vi "Food Truck Main.vi"() -> ()   [LabVIEW 2013]
doc: "This example shows how to debounce a digital signal acquired from a push button switch."
uses:
  <vilib>/Platform/TimedLoop/XDataNode/timing_clust.ctl
  <vilib>/Platform/TimedLoop/XDataNode/nitl_modes.ctl
  <vilib>/Platform/TimedLoop/XDataNode/wakeup.ctl
  Controls/ATT M2X Streams.ctl
  <vilib>/myRIO/Instrument Drivers/Onboard IO/AI/vis/Smart Open.vi
  <vilib>/myRIO/Instrument Drivers/Onboard IO/AI/vis/Read.vi
  <vilib>/myRIO/Instrument Drivers/Onboard IO/DIO/vis/Smart Open.vi
  <vilib>/myRIO/Instrument Drivers/Onboard IO/DIO/vis/Read.vi
  <vilib>/myRIO/Common/Instrument Driver Framework/myRIO v1.0/UART/vis/myRIO v1.0 Close UART.vi
  <vilib>/myRIO/Instrument Drivers/Onboard IO/AI/vis/Open.vi
  <vilib>/myRIO/Instrument Drivers/Onboard IO/DIO/vis/Open.vi
  <vilib>/myRIO/Common/Instrument Driver Framework/myRIO v1.0/AI/vis/myRIO v1.1 Open AI.vi
  <vilib>/myRIO/Common/Instrument Driver Framework/myRIO v1.0/DIO/vis/myRIO v1.1 Open DIO.vi
  <vilib>/myRIO/Common/Instrument Driver Framework/Utilities/vis/Validate Channels.vi
  <vilib>/myRIO/Common/Instrument Driver Framework/myRIO v1.0/AI/vis/myRIO v1.0 Reserve AI.vi
  <vilib>/myRIO/Common/Instrument Driver Framework/myRIO v1.0/DIO/vis/myRIO v1.0 Reserve DIO.vi
  <vilib>/myRIO/Common/Instrument Driver Framework/myRIO v1.0/AI/vis/myRIO v1.0 Build MUX Configuration AI.vi
  <vilib>/myRIO/Common/Instrument Driver Framework/myRIO v1.0/Resource Manager/vis/myRIO v1.0 Reserve Channel List.vi
  <vilib>/myRIO/Common/Instrument Driver Framework/myRIO v1.0/DIO/vis/myRIO v1.0 Build MUX Configuration DIO.vi
  <vilib>/myRIO/Common/Instrument Driver Framework/myRIO v1.0/Resource Manager/vis/myRIO v1.0 Reserve Channel.vi
  <vilib>/myRIO/Common/Instrument Driver Framework/myRIO v1.0/Resource Manager/vis/myRIO v1.0 Unreserve Channel.vi
  <vilib>/myRIO/Common/Instrument Driver Framework/myRIO v1.0/Resource Manager/vis/myRIO v1.0 Create Configuration List.vi
  <vilib>/myRIO/Common/Instrument Driver Framework/myRIO v1.0/Resource Manager/vis/myRIO v1.0 Build Mutex Name.vi
  <vilib>/Instr/_visa.llb/VISA Configure Serial Port (Instr).vi
  <vilib>/myRIO/Common/Instrument Driver Framework/myRIO v1.0/myRIO v1.1 Open.vi
  <vilib>/myRIO/Common/Instrument Driver Framework/myRIO v1.0/AI/vis/myRIO v1.0 Get Scaling Constants AI.vi
  <vilib>/Utility/VariantDataType/GetNumericInfo.vi
  <vilib>/Utility/error.llb/Error Cluster From Error Code.vi
  <vilib>/myRIO/Common/Instrument Driver Framework/Utilities/vis/IO Manager.vi
  <vilib>/myRIO/Common/Instrument Driver Framework/Utilities/vis/Configuration Manager.vi
  <vilib>/myRIO/Common/Instrument Driver Framework/myRIO v1.0/myRIO v1.0 Close.vi
  <vilib>/myRIO/Common/Instrument Driver Framework/myRIO v1.0/AI/vis/myRIO v1.0 Read AI.vi
  <vilib>/LVH/i3 Twitter/SubVIs/Twitter Open - Embedded.vi
  <vilib>/myRIO/Common/Instrument Driver Framework/myRIO v1.0/Resource Manager/vis/myRIO v1.0 Configure IO.vi
  <vilib>/myRIO/Common/Instrument Driver Framework/myRIO v1.0/DIO/vis/myRIO v1.0 Read DIO.vi
  <vilib>/myRIO/Common/Instrument Driver Framework/Utilities/vis/FPGA Ref Manager.vi
  <vilib>/myRIO/Common/Instrument Driver Framework/myRIO v1.0/myRIO v1.0 Reset FPGA.vi
  <vilib>/Platform/TimedLoop/XDataNode/XDataNode.xnode
  <vilib>/Platform/TimedLoop/XDataNode/XDNodeRunTimeDep.lvlib
  <vilib>/LVH/i3 Twitter/i3-twitter.lvlib
  <vilib>/myRIO/Instrument Drivers/Utilities/Utilities.lvlib
panel:
  out "Current Sunshine Value":dbl
  out "Current Food Temp (F)":dbl
  out "Food and Sunshine Timer (30s)":dbl
  out "GPS Timer (180s)":dbl
  out "Latest GPS Transit Data":string
  out "Button Clicks":u16(graph)
  in  "Send to Servers":bool=TRUE
  out "error out":errorcluster
  in  "Stop":bool
  # "Overview: This example shows how to debounce a digital signal acquired from a push button switch.\nInstructions:\n1. Connect an external push button switch to DIO0 on connector A.\n2. Check the myRIO target IP Address in the project and make sure the target IP Address is correct.\n3. Run this VI.\n4. Depending on the quality of the push button switch, you may or may not see jitter."
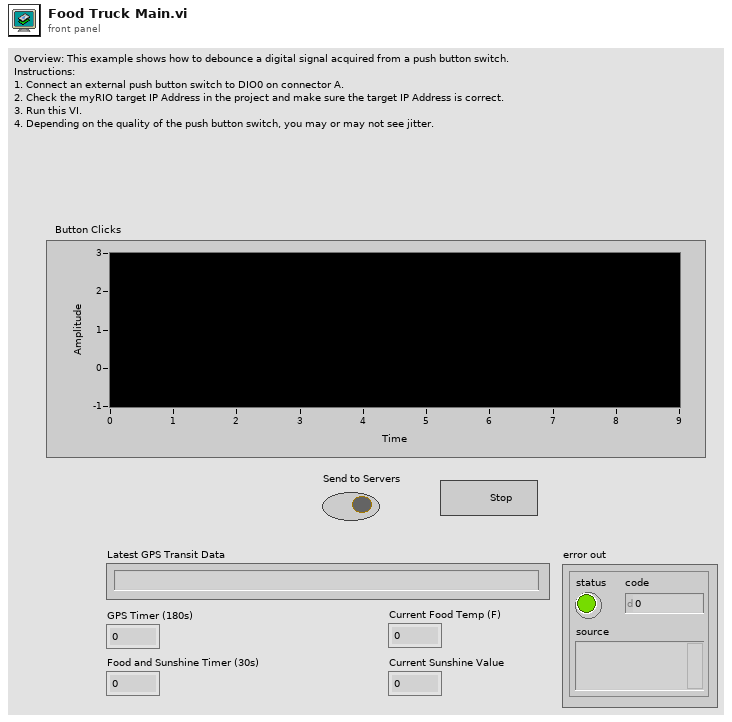
[diagram p1: front panel]
types:
  T1 = cluster{"read mode":enum16{"polling", "blocking"}, "write mode":enum16{"polling", "blocking"}}
  T2 = typedef "ATT M2X Streams.ctl" = enum16{"pay", "deliver", "sunshine", "location", "temp"}
  T3 = typedef "XDNodeRunTimeDep.lvlib/timing_clust.ctl" = cluster{"Expected End [f-1]":u64, "Actual End [f-1]":u64, "Finished Late? [f-1]":bool, "Expected End [i-1]":u64, "Actual End [i-1]":u64, "Finished Late? [i-1]":bool, "Expected Start [i]":u64, "Actual Start [i]":u64, "Expected Start [f]":u64, "Actual Start [f]":u64, "Source Name":string, "Structure Name":string, "Period":i64, "Deadline":i64, "Offset":i64, "Start":i64, "Priority":i32, "Timeout":i32, "Mode":T4, "Wakeup Reason":T5, "Error":errorcluster, "Source Type":string, "Secondary Source Type":string, "Global End Time":u64, "Global Start Time":u64, "Frame Duration":u64, "Iteration Duration":u64, "Assigned CPU":i32, "I/O Scan Engine Mode":u32}
  T4 = typedef "XDNodeRunTimeDep.lvlib/nitl_modes.ctl" = enum32{"No Change", "Process missed periods, maintain original phase", "Discard missed periods, maintain original phase", "Process missed periods, ignore original phase", "Discard missed periods, ignore original phase"}
  T5 = typedef "XDNodeRunTimeDep.lvlib/wakeup.ctl" = enum32{"Normal", "Aborted", "Asynchronous wakeup", "Timing source error", "Timed loop error", "Timeout"}
  T6 = typedef "IMAQ Image.ctl" = refnum<image>
  T7 = typedef "i3-twitter.lvlib/Twitter Handle.ctl" = cluster{"OAuth Credentials":T8, "since ID":string, "max ID":string, "Screen Name":string}
  T8 = typedef "i3-oauth.lvlib/OAuth Handle.ctl" = cluster{"Signature Method":T9, "Version":string, "Client":T10, "Access":T10}
  T9 = typedef "i3-oauth.lvlib/Signature Method.ctl" = enum16{"HMAC-MD5", "HMAC-SHA1", "HMAC-SHA224", "HMAC-SHA256", "HMAC-SHA384", "HMAC-SHA512"}
  T10 = typedef "i3-oauth.lvlib/Credentials.ctl" = cluster{"Token":string, "Secret":string}
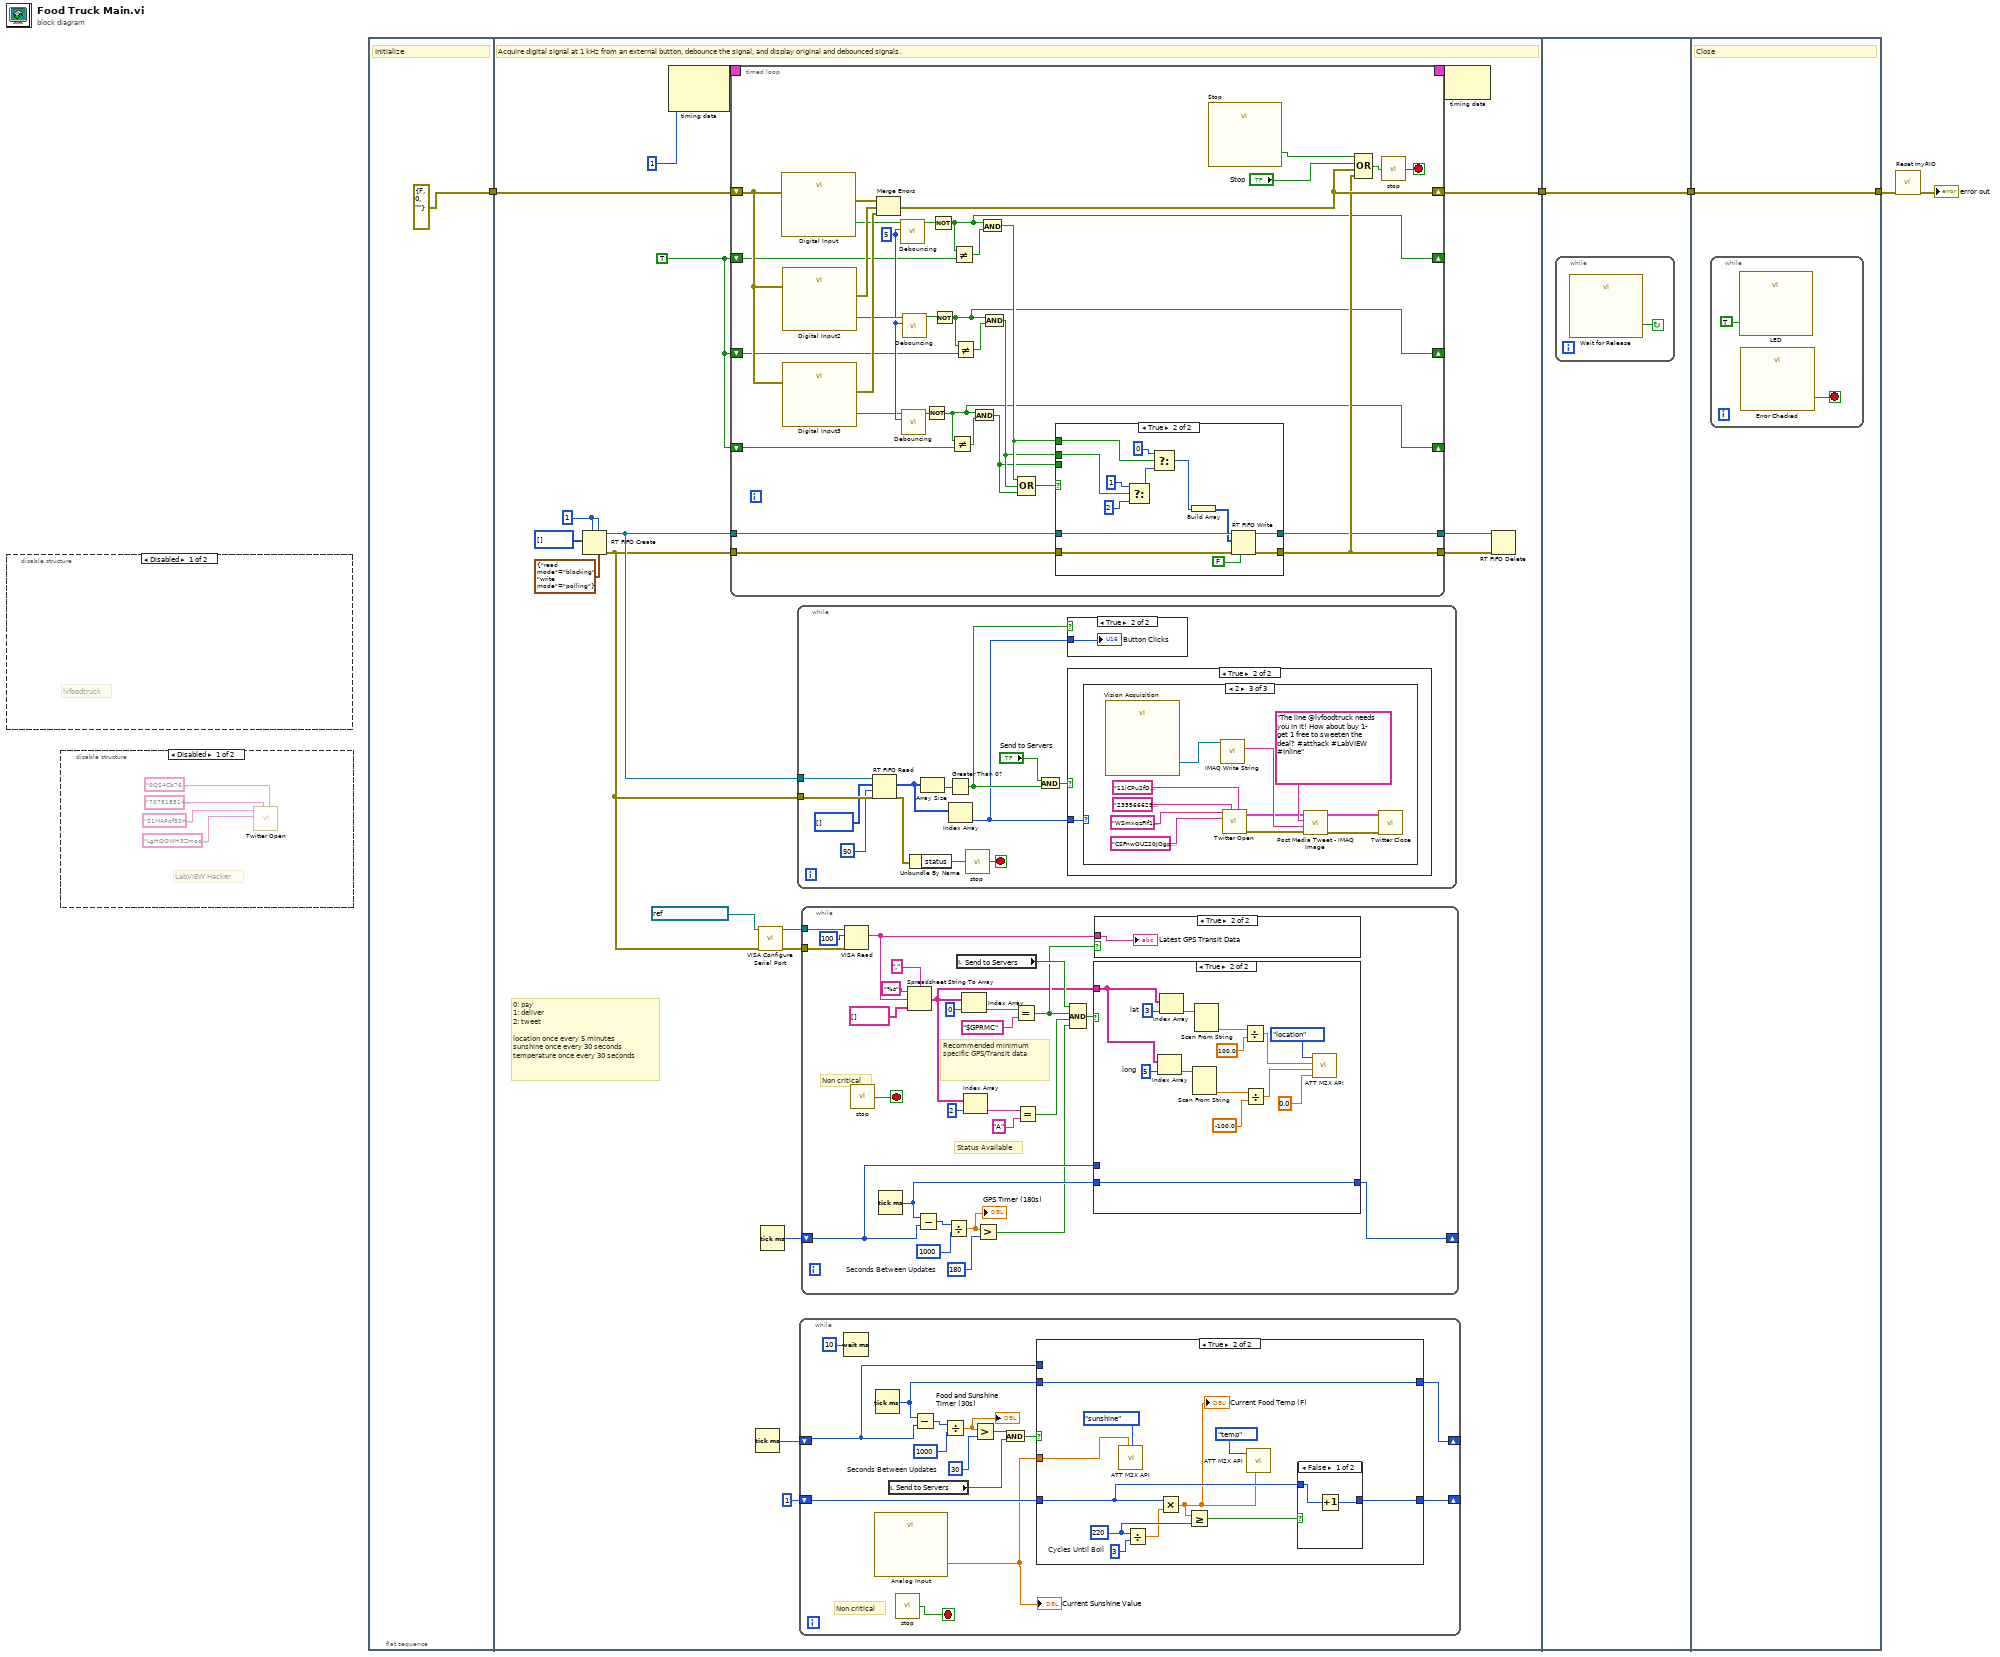
[diagram p0: block diagram]
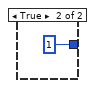
[diagram p5: hidden frame]
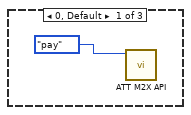
[diagram p10: hidden frame]
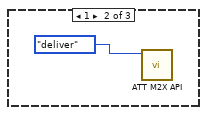
[diagram p11: hidden frame]
diagram:
  n1 = disable-structure shown="Disabled" {
    frame Disabled {
      # "lvfoodtruck"
    }
    frame Enabled {
    }
  }
  n2 = disable-structure shown="Disabled" {
    frame Disabled {
      # "LabVIEW Hacker"
      n3 = call-poly <vilib>:"Twitter Open.vi"("Access Secret"="0QS4Cb76M5wjFwPQ7tOZFvZ8UKrVkLlgPVmxGdh9fF0", "Access Token"="707518514-5GkAQhxzcTAC2kfWjk70QnGtfbYQtNPzzYrLQPwE", "Consumer Secret"="LgHQOWH3ZmoqpZxo5fXh4u8m0SzKCa7qTMPE3lom3I", "Consumer Key"="S1MAPof5SHW02X1IO2gQkA") -> ()  [unwired: 6 in, 2 out]
    }
    frame Enabled {
    }
  }
  n4 = flat-sequence {
    tunnel: [errorcluster {"status"=FALSE, "code"=0, "source"=""} ("error out")] -> w5
    tunnel: w5 -> [w27]
    tunnel: [w26] -> w2
    tunnel: w2 -> [w186]
    tunnel: [w186] -> w1
    tunnel: w1 -> [w188]
    tunnel: [w188] -> w4
    frame #0 {
      # "Initialize"
    }
    frame #1 {
      w18 = TRUE ("A/DIO0 (Pin 11)")
      w24 = u32 1 ("size (10)")
      # "0: pay\n1: deliver\n2: tweet\n\nlocation once every 5 minutes\nsunshine once every 30 seconds\ntemperature once every 30 seconds"
      # "Acquire digital signal at 1 kHz from an external button, debounce the signal, and display original and debounced signals."
      n5 = RT FIFO Create(1:u16[] [], 4:w24, 6:w24, 7:T1 {"read mode"=enum."blocking", "write mode"=enum."polling"} ("r/w modes (polling,polling)")) -> (8:w22:refnum<k33>, 11:w17:errorcluster)  [unwired: 4 in, 1 out]
      n6 = node-c288(i64 1 ("Period")) -> (w29:T3)  [unwired: 1 in]
      n7 = timed-loop {
        shift-right: [w155] -> w26
        shift-left: w27 -> [w157]
        timing: w29 -> [_]
        timing-out: [_] -> w28
        tunnel: w22 -> [w152]
        tunnel: w17 -> [w153]
        tunnel: [w151] -> w19
        tunnel: [w150] -> w20
        shift-right: [w144] -> _
        shift-left: w18 -> [w146]
        shift-right: [w140] -> _
        shift-left: w18 -> [w139]
        shift-right: [w135] -> _
        shift-left: w18 -> [w136]
        stop <- w133 stop-if-true
        w159 = u16 5 ("Cycles to Filter")
        n8 = call "Digital Input"("error in (no error)"=w157) -> ("A/DIO0 (Pin 11)"=w161:bool, "error out"=w156:errorcluster)  [unwired: 25 in]
        n9 = call "Digital Input2"("error in (no error)"=w157) -> ("A/DIO1 (Pin 13)"=w160:bool, "error out"=w164:errorcluster)  [unwired: 25 in]
        n10 = call "Digital Input3"("error in (no error)"=w157) -> ("A/DIO2 (Pin 15)"=w158:bool, "error out"=w163:errorcluster)  [unwired: 25 in]
        n11 = Merge Errors(w156, w164, w163) -> (w155:errorcluster)
        n12 = call "Debouncing.vi"("Cycles to Filter"=w159, "New Input Signal"=w161) -> ("New Signal"=w149:bool)  [unwired: 8 in, 1 out]
        n13 = call "Debouncing.vi"("Cycles to Filter"=w159, "New Input Signal"=w158) -> ("New Signal"=w148:bool)  [unwired: 8 in, 1 out]
        n14 = call "Debouncing.vi"("Cycles to Filter"=w159, "New Input Signal"=w160) -> ("New Signal"=w142:bool)  [unwired: 8 in, 1 out]
        n15 = Not(x=w148) -> (.not. x?=w135:bool)
        n16 = Not(x=w149) -> (.not. x?=w144:bool)
        n17 = Not(x=w142) -> (.not. x?=w140:bool)
        n18 = Not Equal?(x=w135, y=w136) -> (x != y?=w138:bool)
        n19 = Not Equal?(x=w144, y=w146) -> (x != y?=w145:bool)
        n20 = Not Equal?(x=w140, y=w139) -> (x != y?=w143:bool)
        n21 = And(x=w135, y=w138) -> (x .and. y?=w137:bool)
        n22 = And(x=w144, y=w145) -> (x .and. y?=w147:bool)
        n23 = And(x=w140, y=w143) -> (x .and. y?=w141:bool)
        n24 = Compound Arithmetic op=OR(w147, w141, w137) -> (w154:bool)
        n25 = case shown="True" w154 {
          tunnel: w137 -> [_ _]
          tunnel: w141 -> [_ w176]
          tunnel: w147 -> [_ w179]
          tunnel: w153 -> [w165 w173]
          tunnel: w152 -> [w166 w172]
          tunnel: [w165 w170] -> w151
          tunnel: [w166 w169] -> w150
          frame False {
          }
          frame True {
            n26 = Select(t=u16 1 ("size (10)"), s=w176, f=u16 2 ("size (10)")) -> (s? t:f=w177:u16)
            n27 = Select(t=u16 0 ("size (10)"), s=w179, f=w177) -> (s? t:f=w168:u16)
            n28 = Build Array(w168) -> (w167:u16[])
            n29 = RT FIFO Write(0:w172, 1:w167, 3:w173, 5:FALSE ("overwrite on timeout (T)")) -> (8:w169:refnum<k33>, 11:w170:errorcluster)  [unwired: 1 in, 2 out]
          }
        }
        n30 = call "Stop"() -> ("Value"=w132:bool)  [unwired: 26 in, 1 out]
        n31 = Compound Arithmetic op=OR(w132, "Stop", w155, w151) -> (w134:bool)
        n32 = call "stop.vi"("Stop?"=w134) -> ("Stop Called"=w133:bool)
      }
      n33 = Tick Count (ms)() -> (millisecond timer value=w12:u32)
      n34 = call-poly "VISA Configure Serial Port"("VISA resource name"=refnum<visa-resource-name> "ASRL1::INSTR", "error in (no error)"=w17) -> ("VISA resource name out"=w14:refnum<visa-resource-name>, "error out"=w15:errorcluster)  [unwired: 12 in]
      n35 = Tick Count (ms)() -> (millisecond timer value=w13:u32)
      n36 = while {
        tunnel: w22 -> [w116]
        tunnel: w17 -> [w115]
        stop <- w105 stop-if-true
        n37 = RT FIFO Read(0:w116, 1:u16[] [], 2:50 ("timeout in ms (0)"), 3:w115) -> (9:w111:u16[], 11:w106:errorcluster)  [unwired: 3 out]
        n38 = Unbundle By Name(w106) -> ("status"=w104:bool)
        n39 = Array Size(array=w111) -> (size(s)=w112:i32)
        n40 = Greater Than 0?(x=w112) -> (x > 0?=w108:bool)
        n41 = Index Array(array=w111) -> (element=w107:u16)  [unwired: 1 in]
        n42 = call "stop.vi"("Stop?"=w104) -> ("Stop Called"=w105:bool)
        n43 = And(x="Send to Servers", y=w108) -> (x .and. y?=w110:bool)
        n44 = case shown="True" w108 {
          tunnel: w107 -> [_ w117]
          frame False {
          }
          frame True {
            "Button Clicks" <- w117
          }
        }
        n45 = case shown="True" w110 {
          tunnel: w107 -> [_ w118]
          frame False {
          }
          frame True {
            n46 = case shown="2" w118 {
              frame 0, Default {
                n47 = call "ATT M2X API.vi"("M2X Action"=ATT_M2X_Streams."pay") -> ()  [unwired: 11 in]
              }
              frame 1 {
                n48 = call "ATT M2X API.vi"("M2X Action"=ATT_M2X_Streams."deliver") -> ()  [unwired: 11 in]
              }
              frame 2 {
                n49 = call "Vision Acquisition"() -> ("Image Out"=w128:T6)  [unwired: 1 in, 26 out]
                n50 = call-poly "IMAQ Write String"("Image"=w128) -> ("FileString"=w127:string)  [unwired: 8 in, 2 out]
                n51 = call-poly <vilib>:"Twitter Open.vi"("Access Secret"="11iCPu2fD6roKbZOZ3n06jO3pBqYyJw5qbVKj0QqDCqT4", "Access Token"="2355666296-oROjxw2YO7ZtzIdD03PYHHbLc9t4A0mUO1yUdhK", "Consumer Secret"="CSFnwOUZ20JOgpVWiaVuvtkmC6NybXKYc1vpgfGJEs", "Consumer Key"="WSmxqzFIf1JXEhfN34MA") -> ("error out"=w122:errorcluster, "Twitter Handle Out"=w121:T7)  [unwired: 6 in]
                n52 = call "Post Media Tweet - IMAQ Image.vi"("error in"=w122, "PNG String"=w127, "Tweet"="The line @lvfoodtruck needs you in it! How about buy 1- get 1 free to sweeten the deal? #atthack #LabVIEW #Inline", "Twitter Handle In"=w121) -> ("error out"=w130:errorcluster, "Twitter Handle Out"=w129:T7)  [unwired: 6 in]
                n53 = call <vilib>:"Twitter Close.vi"("error in"=w130, "Twitter Handle In"=w129) -> ()  [unwired: 9 in, 1 out]
              }
            }
          }
        }
      }
      n54 = while {
        shift-right: [w37] -> _
        shift-left: w12 -> [w38]
        shift-right: [w34] -> _
        shift-left: u32 1 ("y") -> [w35]
        stop <- w44 stop-if-true
        w43 = u32 30  # Seconds Between Updates
        # "Non critical"
        n55 = Wait (ms)(milliseconds to wait=u32 10) -> ()  [unwired: 1 out]
        n56 = call "Analog Input"() -> ("Sunshine (A/AI0 (Pin 3))"=w30:dbl)  [unwired: 26 in, 1 out]
        "Current Sunshine Value" <- w30
        n57 = Tick Count (ms)() -> (millisecond timer value=w39:u32)
        n58 = local read "Send to Servers"() -> (w31:bool)
        n59 = call "stop.vi"() -> ("Stop Called"=w44:bool)  [unwired: 1 in]
        n60 = Subtract(x=w39, y=w38) -> (x-y=w40:u32)
        n61 = Divide(x=w40, y=u32 1000) -> (x/y=w42:dbl)
        "Food and Sunshine Timer (30s)" <- w42
        n62 = Greater?(x=w42, y=w43) -> (0:w33:bool)
        n63 = And(x=w33, y=w31) -> (x .and. y?=w32:bool)
        n64 = case shown="True" w32 {
          tunnel: w39 -> [_ w49]
          tunnel: w38 -> [w45 _]
          tunnel: [w45 w49] -> w37
          tunnel: w35 -> [w46 w52]
          tunnel: [w46 w53] -> w34
          tunnel: w30 -> [_ w50]
          frame False {
          }
          frame True {
            w56 = u32 3  # Cycles Until Boil
            w57 = u32 220 ("y")
            n65 = call "ATT M2X API.vi"("Sunshine"=w50, "M2X Action"=ATT_M2X_Streams."sunshine") -> ()  [unwired: 10 in]
            n66 = Divide(x=w57, y=w56) -> (x/y=w55:dbl)
            n67 = Multiply(x=w52, y=w55) -> (x*y=w47:dbl)
            "Current Food Temp (F)" <- w47
            n68 = Greater Or Equal?(x=w47, y=w57) -> (x >= y?=w54:bool)
            n69 = call "ATT M2X API.vi"("Food Temp"=w47, "M2X Action"=ATT_M2X_Streams."temp") -> ()  [unwired: 10 in]
            n70 = case shown="False" w54 {
              tunnel: [w59 u32 1 ("y")] -> w53
              tunnel: w52 -> [w58 _]
              frame False {
                n71 = Increment(x=w58) -> (x+1=w59:u32)
              }
              frame True {
              }
            }
          }
        }
      }
      n72 = while {
        tunnel: w15 -> [w85]
        tunnel: w14 -> [w84]
        shift-right: [w61] -> _
        shift-left: w13 -> [w64]
        stop <- w86 stop-if-true
        w65 = u32 180  # Seconds Between Updates
        # "Recommended minimum specific GPS/Transit data"
        # "Status Available"
        # "Non critical"
        n73 = VISA Read(VISA resource name=w84, byte count=u32 100, error in (no error)=w85) -> (read buffer=w73:string)  [unwired: 3 out]
        n74 = call "stop.vi"() -> ("Stop Called"=w86:bool)  [unwired: 1 in]
        n75 = Tick Count (ms)() -> (millisecond timer value=w63:u32)
        n76 = Spreadsheet String To Array(delimiter (Tab)=",", format string="%s", spreadsheet string=w73, array type (2D Dbl)=string[] []) -> (array=w69:string[])
        n77 = Subtract(x=w63, y=w64) -> (x-y=w68:u32)
        n78 = Divide(x=w68, y=u32 1000) -> (x/y=w66:dbl)
        "GPS Timer (180s)" <- w66
        n79 = local read "Send to Servers"() -> (w87:bool)
        n80 = Index Array(array=w69, index=0) -> (element=w74:string)
        n81 = Index Array(array=w69, index=2) -> (element=w75:string)
        n82 = Greater?(x=w66, y=w65) -> (0:w62:bool)
        n83 = Equal?(x=w74, y="$GPRMC") -> (x = y?=w71:bool)
        n84 = Equal?(x=w75, y="A") -> (x = y?=w70:bool)
        n85 = Compound Arithmetic op=AND(w87, w71, w70, w62) -> (w72:bool)
        n86 = case shown="True" w72 {
          tunnel: w69 -> [_ w99]
          tunnel: w64 -> [w89 _]
          tunnel: w63 -> [_ w103]
          tunnel: [w89 w103] -> w61
          frame False {
          }
          frame True {
            w100 = 5  # long
            w101 = 3  # lat
            n87 = Index Array(array=w99, index=w100) -> (element=w92:string)
            n88 = Index Array(array=w99, index=w101) -> (element=w91:string)
            n89 = Scan From String(input string=w92) -> (output 1=w93:dbl)  [unwired: 4 in, 3 out]
            n90 = Scan From String(input string=w91) -> (output 1=w90:dbl)  [unwired: 4 in, 3 out]
            n91 = Divide(x=w90, y=100.0) -> (x/y=w96:dbl)
            n92 = Divide(x=w93, y=-100.0) -> (x/y=w97:dbl)
            n93 = call "ATT M2X API.vi"("elevation"=0.0, "longitude"=w97, "latitude"=w96, "M2X Action"=ATT_M2X_Streams."location") -> ()  [unwired: 8 in]
          }
        }
        n94 = case shown="True" w71 {
          tunnel: w73 -> [_ w88]
          frame False {
          }
          frame True {
            "Latest GPS Transit Data" <- w88
          }
        }
      }
      n95 = node-c288(w28) -> ()  [unwired: 1 out]
      n96 = RT FIFO Delete(0:w20, 3:w19) -> ()  [unwired: 1 in, 1 out]
    }
    frame #2 {
      n97 = while {
        stop <- w187 continue-if-true
        n98 = call "Wait for Release"() -> ("Value"=w187:bool)  [unwired: 26 in, 1 out]
      }
    }
    frame #3 {
      # "Close"
      n99 = while {
        stop <- w189 stop-if-true
        n100 = call "LED"("Error"=TRUE) -> ()  [unwired: 26 in, 1 out]
        n101 = call "Error Checked"() -> ("Value"=w189:bool)  [unwired: 26 in, 1 out]
      }
    }
  }
  n102 = call <vilib>:"Reset myRIO.vi"("error in (no error)"=w4) -> ("error out"=→"error out":errorcluster)  [unwired: 10 in]
